vi "Main_18a not correct.vi"() -> ()   [LabVIEW 2020]
uses:
  RB ENUM_face state.ctl
panel:
  out "MAX":i32
  out "total":i32
  out "number of rows":i32
  in  "Example 2":string="2,2,2\n1,2,2\n3,2,2\n2,1,2\n2,3,2\n2,2,1\n2,2,3\n2,2,4\n2,2,6\n1,2,5\n3,2,5\n2,1,5\n2,3,5"
  out "z":i32
  out "x":i32
  out "y":i32
  out "Array":cluster{"facecube":T1[][][]}[](array[cluster])
  out "Answer":i32
  in  "Puzzle":string="8,17,5\n6,17,7\n8,9,2\n13,5,16\n5,3,9\n19,4,10\n5,14,5\n3,5,12\n4,6,13\n11,9,3\n11,2,14\n3,14,10\n12,1,11\n16,16,13\n1,9,10\n11,9,19\n15,15,12\n10,4,6\n4,12,17\n17,6,15\n19,14,13\n9,13,2\n18,8,14\n17,7,15\n10,5,17\n14,8,17\n11,19,13\n13,3,14\n8,5,10\n8,16,6\n10,7,20\n7,17,5\n12,18,13\n4,8,13\n3,13,13\n4,3,11\n4,9,15\n17,6,7\n13,5,14\n3,12,7\n13,18,7\n1,9,11\n17,8,15\n12,8,2\n4,9,6\n3,7,12\n8,13,4\n3,8,7\n14,7,3\n16,7,14\n17,5,12\n13,8,2\n17,5,5\n16,5,13\n5,4,13\n6,1,9\n1,11,10\n5,13,5\n10,17,5\n6,3,9\n15,6,7\n11,15,17\n18,6,12\n8,3,11\n14,7,14\n10,6,18\n12,11,4\n3,7,15\n7,3,10\n18,8,13\n16,11,19\n11,3,11\n3,15,14\n16,14,3\n19,10,8\n8,13,18\n15,10,3\n20,7,12\n13,15,16\n18,10,9\n10,2,7\n16,5,12\n6,10,18\n12,19,13\n6,5,6\n14,2,8\n4,16,9\n6,17,9\n15,6,5\n9,4,3\n11,7,2\n19,9,6\n14,12,2\n15,6,18\n18,13,7\n5,6,6\n20,11,14\n19,10,10\n18,10,6\n6,10,5\n16,10,18\n3,9,7\n13,2,7\n14,9,19\n9,14,19\n7,18,6\n8,9,19\n11,1,13\n15,17,10\n2,12,13\n5,17,14\n18,9,11\n15,18,15\n7,3,11\n10,18,6\n17,15,14\n17,7,8\n7,3,14\n7,11,19\n7,9,3\n17,11,6\n16,3,10\n9,18,16\n13,1,10\n15,12,16\n14,12,20\n11,2,8\n18,5,9\n11,16,3\n18,10,7\n4,12,6\n5,11,18\n3,14,14\n16,4,12\n8,3,4\n6,14,3\n17,9,18\n2,11,7\n19,15,12\n13,17,15\n10,7,3\n1,11,8\n18,12,16\n18,12,9\n7,4,4\n12,2,7\n7,14,15\n15,13,3\n3,7,11\n12,17,10\n17,5,14\n5,18,11\n5,4,11\n4,15,15\n8,19,12\n18,12,10\n9,3,11\n3,14,12\n18,7,16\n10,9,19\n16,3,11\n15,11,17\n18,7,12\n9,8,19\n3,15,12\n17,4,12\n5,16,7\n8,4,5\n2,7,11\n5,15,17\n9,20,12\n5,11,4\n4,5,9\n4,15,11\n14,14,5\n11,3,6\n12,3,15\n5,6,10\n5,9,5\n18,15,12\n4,12,5\n19,9,15\n4,6,11\n1,14,9\n5,16,15\n9,3,7\n16,10,4\n17,12,7\n18,8,7\n14,5,9\n6,6,14\n5,14,15\n6,7,3\n18,15,15\n12,7,17\n5,14,16\n6,11,3\n6,10,16\n3,7,8\n10,7,4\n8,8,3\n11,4,5\n16,13,18\n13,6,4\n10,17,16\n3,16,10\n10,19,13\n15,5,16\n9,19,6\n9,13,4\n17,16,7\n12,4,15\n7,4,15\n18,17,10\n14,17,7\n13,15,19\n4,10,15\n13,18,17\n14,19,10\n18,10,15\n14,18,8\n16,4,13\n17,14,9\n14,17,5\n6,7,4\n5,9,16\n5,14,17\n14,19,11\n6,18,7\n14,9,18\n17,7,16\n4,10,16\n11,13,3\n3,10,16\n8,9,18\n13,3,15\n17,8,6\n3,13,9\n5,17,10\n14,15,3\n15,5,15\n16,17,15\n9,20,8\n8,2,13\n20,8,8\n17,14,12\n5,7,18\n5,10,16\n3,8,11\n3,11,16\n15,7,5\n17,12,18\n10,19,11\n11,2,10\n18,11,6\n5,11,17\n15,10,15\n18,15,9\n7,5,15\n17,8,5\n5,5,6\n17,14,16\n15,11,5\n8,10,19\n3,13,14\n7,3,9\n13,2,8\n17,9,6\n17,16,11\n11,10,18\n12,17,18\n5,3,14\n12,9,2\n5,14,6\n14,15,15\n15,4,9\n8,12,17\n10,9,3\n4,17,9\n1,11,12\n3,14,11\n11,19,9\n12,17,8\n5,5,9\n19,9,12\n16,4,14\n18,10,14\n8,19,13\n11,3,8\n6,6,4\n13,6,18\n6,14,4\n18,6,8\n4,13,15\n11,7,1\n11,7,18\n10,3,7\n14,15,7\n6,16,9\n14,7,19\n12,6,17\n16,12,5\n3,10,7\n7,12,5\n16,10,15\n17,8,11\n10,18,14\n3,11,4\n7,10,19\n10,4,3\n12,16,6\n9,8,1\n10,4,15\n14,4,5\n5,8,16\n8,13,3\n19,10,9\n17,17,13\n4,5,11\n14,5,16\n16,11,17\n17,7,6\n1,10,11\n11,8,16\n4,15,6\n10,19,14\n6,4,9\n18,11,8\n10,4,5\n11,13,19\n13,6,16\n5,10,17\n3,11,5\n18,17,9\n18,14,11\n10,1,7\n15,9,3\n8,6,3\n6,3,12\n12,2,8\n14,16,17\n16,8,4\n15,7,4\n19,15,9\n17,16,9\n7,14,19\n3,10,8\n9,20,13\n8,8,1\n5,12,4\n8,17,15\n17,3,10\n16,8,6\n18,10,5\n15,8,5\n6,12,4\n1,16,10\n15,17,6\n20,11,11\n4,4,14\n9,9,3\n6,15,17\n16,9,17\n12,12,19\n19,8,10\n4,14,17\n9,15,17\n10,3,14\n4,6,7\n2,8,12\n13,2,11\n7,11,2\n10,19,7\n15,10,2\n6,13,3\n11,10,20\n6,12,18\n15,18,13\n10,8,2\n13,5,5\n11,2,9\n6,17,14\n6,8,5\n14,14,16\n6,8,16\n3,12,16\n8,17,18\n12,2,11\n3,15,11\n10,11,2\n11,17,12\n9,15,3\n6,16,17\n18,6,6\n16,12,16\n7,18,12\n17,15,4\n9,12,18\n17,6,6\n11,8,19\n12,8,3\n20,9,14\n4,12,16\n20,11,10\n4,15,8\n4,7,9\n16,7,5\n10,9,18\n2,11,12\n4,13,16\n9,2,10\n16,7,18\n17,11,16\n6,15,4\n7,18,7\n6,9,19\n8,15,4\n5,16,14\n2,10,7\n8,12,4\n14,18,13\n12,14,17\n15,11,19\n6,13,16\n14,7,18\n19,11,7\n6,17,16\n10,11,3\n7,20,13\n10,18,7\n8,17,6\n4,7,16\n8,3,15\n2,10,9\n5,3,13\n17,10,15\n9,4,6\n8,19,11\n9,16,4\n14,8,19\n13,12,15\n4,13,17\n14,16,5\n5,6,16\n14,13,17\n18,7,13\n12,3,6\n6,4,14\n10,4,9\n3,10,6\n8,19,9\n11,7,19\n19,12,14\n18,9,10\n16,10,17\n16,6,16\n17,15,15\n7,18,11\n1,10,12\n12,4,13\n8,5,5\n20,10,12\n9,18,8\n18,13,9\n8,17,4\n18,7,6\n7,13,4\n15,17,14\n11,17,17\n4,11,16\n7,5,17\n8,15,17\n14,18,6\n15,12,3\n2,7,13\n11,5,5\n19,14,11\n15,18,9\n11,18,5\n7,6,6\n10,11,19\n8,14,3\n6,13,17\n12,5,15\n16,9,3\n3,5,6\n10,4,16\n14,13,19\n3,6,12\n9,15,14\n17,13,7\n7,19,11\n8,14,16\n3,17,12\n9,11,18\n18,14,7\n17,17,9\n8,13,2\n4,16,15\n11,15,4\n8,4,9\n13,6,17\n4,7,12\n13,3,10\n6,5,9\n5,6,5\n15,14,5\n11,4,6\n4,17,13\n3,11,11\n16,13,5\n12,9,1\n13,9,18\n8,17,9\n5,11,15\n16,14,5\n13,11,19\n10,16,17\n9,12,3\n3,12,10\n6,9,4\n5,13,15\n11,6,18\n16,4,9\n7,12,3\n18,12,6\n10,16,18\n14,6,18\n4,5,7\n6,8,18\n15,10,18\n8,3,13\n10,5,18\n3,6,15\n14,6,16\n14,6,17\n12,10,3\n2,14,12\n18,5,10\n15,9,17\n8,6,18\n3,16,14\n10,13,4\n10,15,19\n4,8,17\n13,6,5\n3,6,10\n12,20,10\n11,6,4\n18,4,11\n17,9,11\n15,4,13\n9,17,5\n6,3,11\n11,19,6\n17,6,14\n7,7,18\n8,10,2\n9,3,15\n4,16,13\n11,5,15\n3,6,13\n8,15,18\n14,3,14\n6,5,14\n5,12,18\n8,3,12\n15,4,16\n6,6,15\n16,16,9\n15,3,14\n8,14,18\n10,17,6\n5,9,6\n15,8,16\n18,6,5\n15,13,4\n15,16,5\n10,7,5\n9,7,18\n16,3,13\n4,8,4\n11,11,19\n17,13,12\n17,11,15\n4,13,14\n10,2,6\n4,10,4\n10,3,6\n9,16,17\n8,1,9\n14,20,9\n3,7,14\n8,18,16\n3,11,14\n16,14,15\n3,10,9\n17,12,12\n3,14,5\n10,16,3\n5,15,13\n15,16,7\n12,16,19\n2,12,11\n2,13,10\n13,18,14\n16,15,18\n2,10,15\n2,8,8\n6,7,6\n13,5,17\n6,4,15\n9,17,6\n5,16,13\n11,5,18\n7,17,10\n17,6,5\n14,4,12\n8,12,20\n2,15,10\n18,6,13\n12,19,16\n19,7,5\n19,9,14\n10,13,18\n6,11,19\n10,14,3\n19,7,11\n7,18,16\n14,9,2\n12,4,5\n15,14,6\n5,9,17\n11,14,2\n15,13,18\n16,16,8\n2,5,9\n2,8,10\n16,5,6\n6,18,10\n12,18,15\n4,14,12\n15,8,17\n18,9,9\n11,10,1\n12,3,3\n9,19,9\n8,5,13\n20,14,12\n16,5,15\n1,12,10\n19,15,11\n13,17,10\n12,2,5\n3,5,10\n7,6,5\n5,7,4\n9,6,18\n16,17,12\n7,8,19\n17,11,12\n10,18,15\n13,16,15\n2,12,14\n8,12,2\n14,18,7\n17,5,9\n3,13,5\n10,14,19\n3,8,13\n16,15,3\n11,6,20\n3,14,8\n14,8,18\n7,17,12\n4,13,5\n17,7,5\n8,7,17\n14,4,6\n17,12,4\n13,3,6\n10,12,3\n9,21,11\n17,11,13\n2,16,13\n7,5,3\n14,16,16\n17,15,6\n14,3,13\n11,3,13\n16,16,15\n13,2,13\n17,14,15\n12,2,15\n17,14,11\n10,14,4\n6,8,4\n16,7,15\n11,4,17\n17,17,11\n12,4,17\n6,9,15\n12,9,20\n16,11,5\n18,5,7\n8,11,18\n15,12,6\n12,13,3\n7,15,3\n5,11,3\n11,16,8\n16,17,14\n4,8,7\n14,5,7\n4,13,18\n15,17,7\n16,15,17\n14,20,11\n10,6,14\n12,19,10\n13,3,16\n13,18,8\n13,19,10\n10,10,3\n9,2,8\n6,16,16\n6,16,7\n13,17,5\n3,8,12\n12,13,17\n13,19,12\n19,13,8\n6,10,17\n16,16,7\n7,14,6\n5,15,6\n13,1,12\n7,3,13\n11,17,6\n13,15,3\n10,2,12\n14,2,13\n19,11,6\n8,8,17\n4,6,6\n4,16,10\n4,5,12\n14,19,14\n17,15,16\n11,15,18\n10,15,3\n8,2,10\n15,9,8\n17,13,16\n2,13,14\n15,7,6\n10,12,20\n4,17,14\n12,6,16\n18,7,7\n5,9,4\n16,15,7\n18,16,10\n10,2,10\n13,17,17\n15,6,12\n10,7,2\n11,0,12\n13,2,6\n17,9,5\n10,16,5\n19,10,13\n7,11,16\n5,17,13\n8,18,13\n15,7,19\n3,12,8\n7,18,15\n12,17,3\n16,5,16\n9,16,16\n14,5,15\n8,2,9\n7,16,7\n12,5,16\n19,8,15\n17,10,16\n9,5,6\n12,7,4\n3,4,9\n11,14,19\n12,12,1\n15,12,4\n16,12,17\n18,10,12\n19,12,6\n15,8,15\n12,19,14\n3,8,6\n14,2,12\n11,5,4\n10,5,3\n9,11,3\n7,12,19\n3,5,7\n20,7,11\n15,3,12\n13,4,9\n13,14,2\n17,13,14\n16,4,11\n10,3,17\n15,16,8\n18,16,8\n4,14,14\n11,19,8\n5,11,6\n9,3,16\n10,17,7\n13,9,19\n5,13,8\n12,4,4\n8,13,1\n7,2,11\n6,6,5\n9,5,3\n12,14,3\n14,3,11\n10,6,4\n8,16,18\n10,18,17\n9,7,2\n6,5,8\n10,2,13\n17,8,16\n6,3,10\n7,13,18\n8,18,14\n4,9,17\n12,7,19\n3,12,11\n16,16,14\n4,14,13\n9,5,5\n4,6,16\n7,16,16\n12,15,17\n19,16,11\n8,9,16\n1,13,13\n16,15,5\n2,11,8\n6,2,12\n9,5,15\n12,2,13\n8,13,19\n15,5,7\n7,19,9\n7,1,8\n17,8,4\n5,5,4\n5,4,12\n11,12,3\n8,15,3\n16,16,12\n16,13,17\n5,6,8\n10,10,2\n4,16,14\n10,8,20\n3,9,16\n5,12,5\n7,16,6\n18,6,14\n6,5,17\n2,7,8\n16,17,11\n12,3,12\n11,4,16\n17,11,5\n13,4,11\n15,6,8\n6,10,6\n11,1,10\n10,19,12\n3,14,13\n12,18,9\n7,15,5\n10,3,9\n10,8,18\n16,14,4\n20,9,9\n10,15,2\n10,5,16\n10,17,4\n14,11,2\n15,9,4\n15,3,9\n15,6,17\n2,9,11\n7,13,17\n6,17,15\n16,12,4\n16,5,7\n11,5,17\n5,12,7\n10,3,13\n6,10,4\n17,10,4\n6,4,10\n14,18,14\n12,18,10\n13,18,6\n15,6,13\n15,16,12\n16,6,12\n17,10,7\n17,10,5\n1,9,12\n3,9,5\n17,15,7\n13,13,4\n4,5,13\n15,12,2\n13,4,4\n15,13,17\n19,12,10\n15,18,7\n12,17,17\n16,7,4\n19,7,12\n3,12,5\n11,19,12\n10,20,9\n13,15,18\n18,6,11\n9,1,10\n12,8,20\n18,13,10\n2,12,15\n3,6,11\n14,8,16\n7,10,5\n4,13,6\n10,14,1\n7,12,18\n10,18,11\n2,11,13\n6,6,6\n17,4,8\n13,4,16\n5,14,9\n18,12,5\n4,12,12\n18,15,11\n12,17,4\n17,7,11\n12,17,15\n13,10,1\n2,15,9\n4,10,5\n6,14,6\n15,7,7\n6,16,12\n15,9,2\n12,2,12\n9,4,5\n3,14,7\n9,15,5\n4,7,8\n8,16,17\n19,6,9\n19,8,7\n13,3,9\n14,13,15\n7,17,14\n8,4,12\n13,18,9\n6,5,15\n17,5,6\n13,13,3\n13,17,13\n13,6,2\n11,3,9\n3,8,14\n7,4,8\n4,14,6\n8,5,18\n13,7,18\n13,7,3\n14,11,17\n7,5,16\n13,3,12\n19,12,15\n14,3,5\n17,11,18\n9,3,10\n15,7,3\n2,9,12\n6,18,9\n3,6,9\n13,19,7\n18,11,7\n3,15,8\n2,12,12\n16,15,11\n4,4,11\n6,7,11\n1,10,13\n15,3,11\n14,18,10\n6,9,18\n18,9,15\n12,19,11\n7,6,7\n3,12,18\n3,11,9\n14,17,6\n16,16,11\n18,14,14\n8,20,11\n18,6,7\n15,6,16\n5,9,3\n14,2,14\n10,7,18\n7,4,17\n20,6,9\n15,5,10\n15,4,12\n20,10,15\n6,12,2\n10,4,4\n5,15,15\n5,16,10\n6,11,2\n10,13,2\n7,15,4\n15,16,4\n16,5,8\n4,6,15\n8,5,14\n4,17,12\n6,14,5\n11,17,7\n15,14,15\n17,12,5\n6,18,13\n16,17,9\n7,7,16\n4,6,9\n7,10,3\n16,14,12\n19,12,12\n15,17,9\n13,2,12\n6,9,3\n12,3,9\n15,14,3\n14,14,19\n14,8,3\n9,8,18\n4,13,7\n10,4,8\n8,1,7\n5,5,13\n14,3,16\n6,20,9\n6,15,18\n5,14,18\n19,9,8\n5,2,12\n16,8,15\n10,3,8\n13,15,4\n8,16,3\n13,13,2\n14,18,12\n16,5,14\n11,14,18\n5,7,5\n8,9,20\n9,8,3\n16,16,6\n13,20,9\n11,18,14\n15,13,5\n11,14,17\n12,17,6\n10,17,15\n6,8,15\n2,7,12\n12,20,13\n9,14,17\n12,16,5\n10,19,6\n7,7,4\n1,11,11\n19,6,10\n15,14,4\n19,13,12\n4,7,6\n9,2,12\n9,19,15\n18,14,16\n11,10,2\n13,16,4\n17,12,15\n2,10,10\n2,13,13\n5,10,3\n10,16,7\n11,19,10\n17,14,8\n12,12,20\n7,5,8\n11,8,20\n5,15,8\n3,9,8\n13,5,13\n17,15,10\n14,11,19\n15,5,4\n15,3,8\n15,4,6\n4,15,14\n17,11,17\n12,6,15\n3,16,7\n4,11,5\n13,10,3\n7,14,3\n6,17,12\n14,16,4\n4,16,12\n4,14,5\n14,19,9\n19,13,9\n10,10,19\n11,11,1\n18,16,12\n17,17,8\n10,12,2\n7,18,8\n1,8,12\n19,8,6\n4,6,8\n13,14,17\n20,10,8\n19,7,7\n12,3,14\n2,9,8\n5,17,11\n11,8,2\n7,18,9\n8,7,3\n9,15,18\n10,6,16\n7,16,3\n15,8,18\n11,14,3\n17,13,6\n11,8,18\n14,5,5\n17,16,14\n17,13,4\n9,7,17\n13,5,6\n14,3,12\n3,13,16\n11,3,7\n16,10,16\n11,16,4\n7,3,15\n5,16,11\n20,9,10\n18,8,9\n19,8,8\n20,9,13\n11,16,16\n15,11,2\n1,13,12\n14,13,4\n12,18,11\n14,16,3\n11,5,11\n17,7,13\n15,11,18\n7,17,9\n5,5,14\n11,9,2\n4,7,14\n7,17,15\n5,12,17\n3,8,15\n18,10,16\n15,4,11\n12,5,6\n19,11,11\n11,18,17\n18,13,16\n7,4,7\n7,5,6\n13,10,19\n13,18,10\n16,15,16\n5,7,15\n12,12,2\n2,14,8\n20,9,11\n4,7,11\n5,11,12\n16,16,10\n3,17,9\n2,9,9\n17,18,9\n3,12,15\n5,3,11\n15,4,15\n20,10,14\n19,13,11\n5,13,18\n17,9,4\n13,12,17\n3,15,13\n14,10,6\n16,16,5\n5,8,17\n15,3,6\n18,15,10\n15,6,6\n18,11,14\n17,12,13\n4,6,14\n5,14,3\n15,5,6\n11,15,3\n12,2,9\n14,3,15\n17,12,16\n15,17,13\n13,12,1\n14,3,10\n18,9,14\n12,17,11\n16,11,15\n18,8,6\n3,12,6\n3,9,6\n7,16,8\n16,12,15\n18,8,10\n4,5,10\n12,19,7\n14,2,9\n8,7,6\n12,3,11\n4,7,7\n9,18,14\n4,6,5\n11,17,16\n8,19,10\n12,8,19\n3,17,13\n15,12,18\n4,4,13\n10,19,8\n16,8,17\n9,7,16\n19,14,9\n9,8,2\n16,8,13\n7,5,14\n7,6,4\n18,11,10\n6,4,5\n18,7,14\n18,11,13\n9,6,3\n8,16,15\n7,8,3\n12,9,3\n9,19,7\n8,6,16\n10,4,17\n17,4,14\n11,13,18\n6,8,17\n3,7,17\n16,4,8\n2,10,8\n5,18,8\n9,3,6\n18,9,5\n9,15,19\n3,16,9\n7,6,17\n7,16,17\n12,11,19\n12,10,2\n4,7,10\n6,19,13\n19,11,10\n9,10,1\n12,14,4\n4,9,4\n18,16,9\n5,3,8\n9,18,4\n3,13,6\n16,15,14\n13,8,19\n12,16,14\n8,10,15\n11,21,12\n5,15,5\n8,9,15\n18,11,5\n16,17,8\n10,17,17\n11,8,3\n7,19,12\n14,16,8\n17,15,12\n11,11,4\n7,6,19\n3,16,12\n17,5,10\n11,3,16\n8,15,14\n8,15,5\n2,9,13\n5,11,5\n4,4,8\n12,5,17\n7,5,7\n6,19,11\n4,7,4\n17,9,7\n15,7,16\n9,14,3\n14,4,15\n16,7,17\n3,12,9\n17,9,16\n8,18,10\n11,16,5\n10,18,8\n14,5,6\n12,15,16\n10,6,19\n14,7,17\n2,14,11\n8,5,8\n16,9,4\n8,3,7\n8,3,14\n19,9,13\n6,8,3\n17,14,17\n13,3,13\n4,13,4\n3,10,14\n17,16,12\n17,5,11\n12,3,10\n15,8,3\n17,9,14\n14,7,4\n5,9,18\n10,2,9\n13,4,7\n7,15,17\n11,13,20\n8,18,7\n12,13,20\n17,16,13\n10,6,2\n3,6,5\n7,2,13\n12,4,16\n14,15,18\n12,9,17\n8,12,18\n7,10,2\n17,3,8\n9,3,9\n14,9,3\n10,3,10\n14,6,5\n16,14,10\n6,3,13\n9,19,12\n19,9,11\n9,9,19\n17,15,13\n19,6,13\n10,3,12\n15,4,14\n10,5,5\n6,12,16\n10,11,18\n4,9,5\n19,15,8\n4,15,7\n14,16,14\n12,1,9\n9,14,2\n12,15,3\n14,10,17\n15,15,17\n14,4,10\n3,13,12\n17,17,10\n9,17,4\n3,9,11\n11,15,13\n20,11,8\n18,13,13\n3,11,8\n14,3,7\n18,11,12\n19,14,8\n18,13,6\n10,16,16\n9,1,12\n5,8,13\n11,2,13\n2,15,8\n11,3,14\n8,17,14\n8,6,6\n5,13,4\n5,15,4\n4,3,7\n14,17,14\n12,15,2\n13,5,4\n14,15,4\n15,14,16\n19,12,9\n19,8,11\n7,11,3\n3,5,13\n6,13,19\n15,13,6\n11,6,17\n18,8,8\n11,18,10\n10,12,18\n2,10,12\n18,9,17\n18,7,8\n7,16,11\n9,20,11\n17,13,17\n9,14,1\n4,4,12\n6,19,10\n2,9,14\n18,11,11\n18,5,13\n3,7,13\n13,12,2\n13,17,6\n2,7,9\n18,8,11\n4,16,11\n7,7,5\n14,17,16\n12,3,5\n11,17,18\n15,16,16\n9,13,19\n17,14,14\n6,17,6\n13,4,5\n5,8,18\n9,11,20\n17,10,8\n8,16,2\n17,7,7\n14,14,17\n15,7,14\n14,10,19\n6,11,5\n15,8,4\n9,3,14\n5,14,4\n4,11,4\n15,16,11\n7,16,14\n8,18,12\n17,12,6\n6,9,17\n13,15,17\n4,4,9\n8,7,18\n12,19,9\n16,14,17\n2,7,7\n7,14,18\n18,12,15\n5,17,9\n6,2,9\n12,19,15\n5,7,17\n16,15,15\n13,3,11\n8,2,11\n11,4,8\n10,12,21\n9,15,16\n3,7,9\n10,2,11\n4,8,6\n17,10,6\n11,3,17\n4,11,18\n11,4,3\n4,11,8\n18,5,8\n12,13,2\n14,4,4\n13,11,18\n8,14,2\n6,7,16\n20,11,13\n12,3,7\n4,11,10\n6,3,6\n12,18,7\n8,5,11\n15,2,11\n17,5,7\n18,14,9\n9,4,11\n13,11,3\n10,19,10\n18,14,8\n16,11,4\n10,4,11\n10,8,19\n13,18,5\n10,9,1\n13,20,10\n6,8,6\n10,14,2\n18,8,5\n9,14,18\n3,8,8\n16,9,16\n17,8,14\n9,6,16\n7,9,20\n3,13,11\n17,8,13\n18,10,4\n16,6,9\n12,19,8\n6,15,6\n8,8,4\n7,14,4\n13,17,14\n19,6,6\n4,17,11\n8,17,16\n12,9,19\n2,11,11\n19,8,13\n6,5,5\n9,17,16\n14,4,9\n17,8,9\n4,13,9\n2,8,13\n17,4,10\n13,8,16\n2,13,11\n5,5,11\n15,9,19\n11,15,19\n7,17,18\n7,3,7\n13,16,16\n8,17,12\n15,2,14\n9,9,2\n7,4,13\n7,18,14\n5,16,5\n17,16,8\n11,1,7\n4,11,13\n18,11,9\n4,15,10\n2,7,10\n12,10,18\n7,10,16\n14,3,6\n20,10,11\n4,8,11\n6,15,5\n3,12,13\n5,4,10\n2,9,7\n16,5,9\n13,5,3\n15,7,17\n6,16,11\n9,18,15\n10,20,10\n13,8,18\n19,10,12\n5,6,17\n17,10,3\n15,11,3\n18,12,11\n13,4,6\n13,14,16\n2,12,10\n6,14,18\n15,16,6\n10,18,10\n4,14,16\n3,13,7\n13,8,20\n10,18,5\n12,2,10\n18,5,11\n15,2,6\n13,7,2\n10,3,15\n10,15,16\n4,6,12\n20,12,7\n8,3,10\n16,4,10\n20,13,8\n17,3,12\n13,11,4\n8,3,8\n7,3,6\n5,17,8\n18,13,11\n14,11,16\n5,11,16\n11,16,6\n16,9,5\n4,3,9\n14,4,16\n5,10,4\n7,2,10\n14,4,8\n14,17,9\n4,5,15\n15,15,5\n6,17,8\n5,3,12\n3,14,9\n8,12,19\n5,7,11\n18,7,15\n9,5,2\n13,10,17\n7,9,18\n19,7,13\n3,7,6\n13,9,2\n4,10,13\n10,14,17\n3,12,12\n12,7,18\n16,6,7\n15,8,19\n9,15,4\n12,7,2\n14,13,18\n6,4,11\n3,7,5\n18,9,13\n17,3,11\n5,4,15\n9,16,3\n13,10,2\n16,19,10\n19,14,10\n13,2,14\n9,3,13\n12,18,12\n15,18,12\n10,20,14\n6,7,18\n13,8,3\n6,11,20\n8,4,10\n11,3,10\n5,6,13\n8,2,12\n2,9,10\n3,12,14\n2,12,7\n18,6,15\n15,13,19\n16,15,9\n17,5,8\n7,6,18\n7,2,7\n19,7,9\n17,6,12\n6,19,14\n5,16,17\n6,10,3\n7,12,4\n17,15,11\n12,8,18\n2,14,13\n5,8,6\n15,4,10\n7,7,17\n19,9,9\n16,14,8\n16,7,13\n11,10,3\n14,11,1\n16,15,12\n5,15,7\n7,3,8\n12,3,13\n11,3,15\n9,3,5\n13,2,10\n19,11,9\n11,12,20\n8,8,2\n7,9,19\n19,13,14\n18,9,6\n18,15,14\n5,6,14\n20,5,9\n8,4,15\n8,16,5\n2,6,11\n8,4,4\n6,19,9\n7,18,10\n14,8,4\n9,18,7\n9,6,19\n9,5,16\n18,15,7\n16,16,16\n8,12,3\n5,16,9\n5,6,15\n15,6,4\n8,2,14\n9,13,1\n2,14,7\n11,16,2\n9,18,6\n18,9,16\n17,15,8\n6,13,14\n14,4,11\n9,12,2\n11,16,18\n9,4,9\n15,15,6\n9,8,17\n5,12,6\n16,8,3\n15,14,2\n6,18,14\n18,16,14\n14,7,6\n16,3,9\n15,6,14\n10,15,18\n7,5,4\n12,3,16\n9,6,14\n6,18,15\n18,15,8\n6,15,7\n16,3,8\n2,13,8\n9,16,5\n8,7,16\n18,11,17\n17,9,17\n17,8,17\n17,12,17\n16,6,6\n8,11,3\n5,13,14\n8,2,8\n15,17,11\n5,6,9\n2,11,9\n11,2,11\n5,18,12\n18,16,11\n6,9,8\n12,5,4\n1,8,8\n6,14,17\n12,8,1\n13,3,7\n2,10,13\n7,13,3\n17,14,13\n15,18,14\n7,17,7\n13,15,2\n9,2,13\n6,2,10\n6,14,14\n15,14,12\n8,2,15\n13,11,2\n4,15,13\n18,12,14\n16,17,7\n20,10,9\n16,15,6\n12,11,3\n6,18,12\n11,4,4\n18,11,16\n17,12,9\n3,8,5\n7,4,6\n13,4,13\n18,9,7\n15,5,12\n2,13,12\n14,3,9\n3,6,8\n16,8,11\n11,12,18\n19,12,13\n16,15,4\n13,16,6\n4,9,7\n12,9,5\n15,7,18\n15,10,5\n19,5,10\n10,2,8\n10,4,14\n17,4,11\n19,14,12\n3,11,13\n8,18,9\n1,10,9\n6,4,7\n12,7,3\n2,15,11\n13,19,11\n14,17,10\n2,5,12\n11,20,10\n4,7,17\n10,17,8\n7,11,18\n4,10,17\n13,12,20\n7,8,4\n19,13,13\n4,5,8\n13,6,19\n5,12,3\n5,16,6\n13,4,12\n9,11,2\n15,15,2\n5,16,8\n8,3,16\n13,4,15\n14,12,4\n13,16,5\n14,15,5\n4,7,5\n6,4,13\n11,18,8\n12,17,5\n7,2,9\n14,2,11\n10,10,20\n9,10,20\n17,15,9\n12,14,18\n8,11,19\n19,7,14\n10,13,19\n12,10,19\n6,20,11\n5,8,15\n7,2,8\n9,12,20\n8,13,16\n2,14,6\n3,10,5\n16,7,6\n7,2,12\n6,16,6\n13,7,4\n14,9,17\n9,19,8\n3,5,11\n17,4,9\n16,15,8\n10,5,6\n9,1,9\n6,4,16\n19,12,11\n6,9,5\n11,17,10\n10,19,15\n9,15,2\n3,17,8\n20,13,11\n15,4,7\n7,17,16\n8,16,7\n18,9,12\n3,10,12\n4,14,10\n4,5,14\n4,6,10\n15,17,15\n11,11,3\n12,2,14\n9,7,3\n9,3,8\n13,20,13\n4,12,4\n8,4,7\n16,6,10\n19,10,7\n6,3,15\n5,7,16\n9,1,15\n8,1,11\n4,8,15\n8,11,20\n8,16,4\n13,1,9\n11,6,3\n6,11,4\n15,16,14\n5,4,14\n10,20,11\n14,2,10\n19,11,12\n18,12,13\n7,10,18\n3,14,15\n4,12,9\n5,8,4\n8,20,9\n13,5,15\n14,19,13\n18,9,8\n10,12,19\n4,13,11\n4,18,14\n16,5,10\n12,4,6\n16,8,8\n6,5,4\n11,4,18\n7,4,9\n9,5,17\n17,9,15\n16,12,12\n16,18,9\n5,5,10\n3,5,8\n4,10,14\n6,15,16\n8,1,10\n17,14,10\n15,10,4\n11,9,20\n5,7,3\n13,7,16\n12,10,20\n18,10,10\n4,10,10\n7,4,3\n15,9,18\n11,12,4\n8,10,17\n4,19,10\n8,19,8\n16,9,2\n11,2,7\n11,7,17\n10,8,3\n9,11,19\n7,13,2\n11,17,4\n10,12,1\n5,5,8\n13,13,19\n16,18,15\n6,16,8\n15,17,16\n15,10,17\n13,15,15\n11,3,12\n13,12,18\n7,16,5\n12,11,1\n19,7,10\n7,3,12\n19,12,7\n18,16,7\n13,14,3\n15,13,2\n8,6,4\n8,6,15\n5,14,11\n3,9,14\n8,5,4\n14,12,16\n19,8,12\n10,7,19\n9,16,18\n11,18,13\n15,16,17\n3,9,13\n10,13,1\n16,13,4\n8,11,1\n14,5,3\n12,6,18\n18,8,15\n11,18,11\n4,14,8\n5,12,15\n2,8,9\n3,10,13\n6,12,17\n3,6,14\n8,7,4\n16,8,18\n4,5,5\n4,8,9\n16,19,11\n13,3,8\n6,6,17\n4,12,13\n8,17,17\n10,13,3\n16,16,4\n12,6,5\n7,19,13\n18,14,12\n14,6,3\n17,7,12\n17,16,10\n2,12,9\n1,12,12\n11,13,17\n15,17,8\n11,3,5\n14,4,14\n9,4,13\n12,16,17\n5,17,7\n18,4,10\n12,18,5\n3,15,10\n9,10,19\n6,10,2\n10,6,1\n6,12,3\n13,4,17\n15,15,16\n5,15,12\n15,15,14\n11,2,5\n12,5,3\n14,18,11\n15,16,15\n11,19,7\n3,11,7\n5,9,14\n9,1,13\n15,18,11\n14,12,3\n11,20,9\n2,13,15\n4,18,12\n10,4,7\n19,13,10\n11,20,12\n9,8,16\n12,18,14\n9,18,13\n12,16,15\n17,5,13\n11,2,6\n9,4,17\n7,17,13\n11,6,15\n18,13,14\n9,17,15\n12,11,2\n16,17,13\n6,16,4\n14,14,3\n19,10,11\n16,6,5\n10,18,4\n6,13,2\n18,9,4\n10,9,2\n13,16,17\n13,18,15\n7,17,11\n6,13,4\n1,12,13\n11,1,12\n18,14,10\n7,19,14\n10,3,16\n10,21,12\n15,19,10\n9,13,3\n13,7,17\n8,11,2\n6,5,7\n6,13,5\n13,17,8\n15,4,8\n19,10,6\n2,11,6\n10,19,9\n5,4,7\n10,17,13\n6,13,18\n8,7,19\n2,12,8\n9,2,6\n12,6,19\n13,12,3\n7,4,11\n3,13,17\n10,2,5\n20,7,8\n14,4,7\n13,17,4\n14,18,15\n15,6,15\n8,17,8\n3,9,9\n17,18,7\n5,7,7\n3,11,12\n17,6,13\n4,11,7\n17,8,18\n5,14,14\n5,6,4\n6,18,11\n17,3,13\n3,13,8\n5,7,6\n1,13,10\n5,13,16\n19,7,8\n4,11,17\n6,17,13\n15,17,5\n18,13,8\n18,8,16\n1,8,13\n4,9,12\n12,15,18\n7,13,5\n9,18,17\n11,6,16\n13,4,14\n9,4,4\n10,17,14\n13,14,18\n12,15,19\n6,12,6\n7,19,10\n1,12,9\n20,10,13\n14,14,15\n12,15,4\n4,12,15\n5,10,18\n10,8,17\n6,6,3\n3,10,10\n5,18,7\n7,12,17\n8,15,2\n12,14,20\n11,16,17\n4,14,15\n13,20,8\n4,11,14\n7,16,15\n9,19,14\n9,6,20\n3,16,8\n10,1,8\n11,13,1\n14,1,11\n16,18,10\n1,11,9\n14,20,10\n9,19,13\n10,20,12\n3,14,16\n19,6,11\n18,11,15\n19,13,7\n8,18,6\n17,6,16\n16,13,15\n14,15,2\n13,1,8\n6,4,8\n17,6,10\n1,8,10\n15,16,13\n8,19,6\n2,8,11\n7,10,1\n4,16,6\n19,10,15\n19,16,9\n9,10,18\n16,17,6\n16,10,19\n12,1,10\n15,5,5\n2,6,8\n19,8,14\n4,18,11\n10,11,1\n10,21,10\n6,6,16\n5,5,7\n9,5,18\n8,10,3\n12,18,16\n9,2,7\n9,18,5\n5,4,6\n10,11,20\n9,19,11\n12,19,12\n3,11,10\n15,3,13\n7,17,6\n20,11,9\n11,8,17\n11,11,2\n7,4,10\n18,10,8\n13,13,18\n6,8,19\n18,14,15\n6,19,12\n15,12,5\n18,7,9\n8,12,1\n18,6,10\n3,12,4\n10,13,20\n17,15,5\n3,7,7\n7,14,2\n8,4,16\n11,10,21\n11,12,2\n14,19,12\n2,12,6\n16,10,8\n8,17,7\n6,7,5\n11,12,1\n7,13,16\n3,5,14\n12,20,8\n2,10,14\n4,12,7\n8,16,16\n7,4,16\n8,19,16\n9,1,11\n2,10,11\n10,12,17\n19,11,13\n17,14,6\n11,17,15\n3,15,9\n13,19,8\n6,17,10\n12,3,8\n4,4,10\n16,18,6\n6,16,5\n14,4,13\n7,3,17\n16,14,7\n2,16,12\n5,12,16\n6,17,11\n7,10,15\n15,11,4\n10,16,4\n19,11,14\n4,16,8\n6,9,2\n6,16,15\n18,14,6\n7,1,10\n6,5,13\n17,13,15\n20,13,14\n8,9,3\n16,14,11\n17,13,8\n4,17,10\n2,14,9\n8,3,9\n6,15,15\n19,6,8\n4,4,7\n16,3,14\n9,14,16\n4,10,7\n13,3,17\n16,9,18\n9,2,14\n5,17,5\n14,6,2\n15,2,13\n14,17,15\n7,16,12\n10,4,10\n14,19,8\n9,17,7\n6,9,6\n9,12,19\n12,4,18\n15,11,6\n14,5,17\n17,13,10\n9,19,10\n13,2,9\n12,13,19\n15,2,12\n8,14,4\n5,17,12\n19,9,10\n12,6,3\n15,3,5\n9,6,5\n4,12,8\n12,13,18\n8,5,16\n8,4,14\n13,11,20\n14,13,2\n7,12,7\n9,1,7\n15,16,9\n9,9,20\n5,15,14\n12,10,1\n14,17,8\n8,11,17\n10,18,13\n9,4,7\n14,18,9\n12,19,5\n12,1,8\n9,13,18\n5,7,12\n18,6,16\n3,8,9\n18,15,17\n1,10,14\n12,16,4\n14,7,16\n18,10,11\n7,1,13\n14,7,2\n18,13,15\n16,13,16\n11,5,3\n9,5,4\n14,12,18\n12,13,1\n18,15,13\n2,6,10\n4,17,6\n12,1,12\n4,16,7\n12,16,16\n8,18,15\n14,10,18\n9,9,0\n10,1,13\n9,6,4\n12,6,9\n7,7,3\n9,17,14\n17,14,7\n5,18,9\n12,0,11\n16,11,18\n7,14,16\n14,10,3\n13,12,4\n1,11,6\n13,18,11\n3,6,7\n3,15,7\n3,16,13\n19,12,8\n11,15,6\n12,4,8\n8,7,2\n8,10,18\n3,4,13\n7,6,14\n6,12,5\n20,8,12\n3,9,15\n13,14,4\n16,5,5\n5,4,8\n18,15,6\n7,15,18\n7,13,19\n11,8,4\n12,12,17\n14,5,8\n6,7,2\n14,9,20\n16,10,3\n19,11,8\n13,16,18\n15,4,17\n20,12,9\n11,18,16\n5,10,19\n1,9,13\n10,6,17\n3,9,12\n12,17,7\n16,11,6\n5,17,15\n18,13,12\n3,15,15\n10,3,11\n16,5,4\n20,14,11\n5,10,14\n13,17,16\n12,1,13\n10,4,13\n5,5,16\n11,8,1\n16,4,15\n16,17,16\n6,19,8\n11,6,2\n4,18,10\n6,6,7\n14,11,18\n17,10,18\n11,4,13\n14,12,17\n5,16,12\n2,9,6\n12,4,14\n1,14,11\n13,17,3\n5,18,10\n13,15,6\n11,1,9\n11,20,11\n17,10,14\n14,11,3\n14,9,4\n4,3,8\n14,12,5\n12,12,4\n2,6,9\n8,14,19\n4,7,13\n14,12,19\n4,14,7\n18,6,9\n11,12,17\n13,6,3\n12,7,16\n11,2,15\n18,7,5\n5,9,19\n1,8,9\n12,14,16\n5,15,16\n16,18,13\n11,18,9\n15,9,15\n7,5,13\n17,6,8\n17,7,10\n11,18,15\n10,7,1\n2,8,6\n11,13,2\n5,6,11\n7,16,10\n6,5,10\n7,8,2\n8,6,19\n3,13,10\n18,11,4\n17,3,15\n17,11,8\n9,16,6\n15,3,15\n8,5,17\n7,15,8\n15,13,16\n17,4,13\n15,9,16\n16,12,11\n17,12,11\n6,15,13\n2,8,15\n17,7,14\n8,4,6\n17,11,3\n11,20,8\n11,17,14\n8,8,19\n1,12,14\n14,17,11\n7,16,4\n12,14,19\n11,15,20\n8,5,9\n12,11,17\n16,14,6\n11,5,16\n17,9,3\n16,11,16\n3,7,10\n15,3,7\n13,12,5\n7,14,17\n20,12,12\n11,15,2\n3,11,15\n6,12,7\n7,14,5\n17,13,18\n8,5,6\n7,17,4\n4,9,16\n15,18,6\n14,17,17\n10,14,18\n9,4,10\n16,6,11\n11,18,7\n17,12,14\n13,19,6\n14,14,4\n10,20,13\n6,5,11\n7,12,2\n8,15,16\n3,10,11\n4,11,15\n4,9,14\n4,9,10\n10,5,19\n9,2,11\n15,10,19\n10,18,9\n9,9,18\n16,14,16\n4,13,3\n19,11,15\n19,13,16\n16,6,14\n7,2,14\n8,19,7\n16,4,7\n12,11,20\n16,12,18\n10,8,4\n10,5,15\n20,8,13\n4,18,7\n16,6,15\n14,11,4\n10,2,16\n8,8,20\n14,9,16\n7,6,3\n4,8,14\n10,20,8\n7,13,8\n7,17,17\n14,17,12\n2,8,7\n14,2,6\n15,14,17\n4,8,10\n18,5,12\n5,5,15\n11,7,4\n6,18,8\n17,8,3\n7,6,2\n5,14,7\n9,1,14\n10,11,5\n13,18,13\n1,7,12\n8,4,17\n8,18,11\n17,6,11\n12,13,4\n16,4,6\n3,4,11\n5,14,12\n16,18,7\n11,17,13\n9,7,4\n17,13,3\n13,15,5\n8,17,13\n14,8,20\n2,8,14\n15,3,16\n12,19,6\n7,7,19\n6,7,19\n11,10,19\n5,19,9\n7,5,5\n7,9,17\n7,8,17\n16,6,8\n14,16,18\n16,10,7\n4,15,12\n13,20,11\n10,15,4\n14,17,13\n2,15,14\n10,15,17\n7,9,1\n10,17,11\n16,6,13\n17,16,15\n13,17,11\n17,14,5\n7,11,4\n13,5,7\n7,6,16\n14,9,1\n16,15,13\n15,5,14\n3,11,6"
  in  "Example":string="2,2,2\n1,2,2\n3,2,2\n2,1,2\n2,3,2\n2,2,1\n2,2,3\n2,2,4\n2,2,6\n1,2,5\n3,2,5\n2,1,5\n2,3,5"
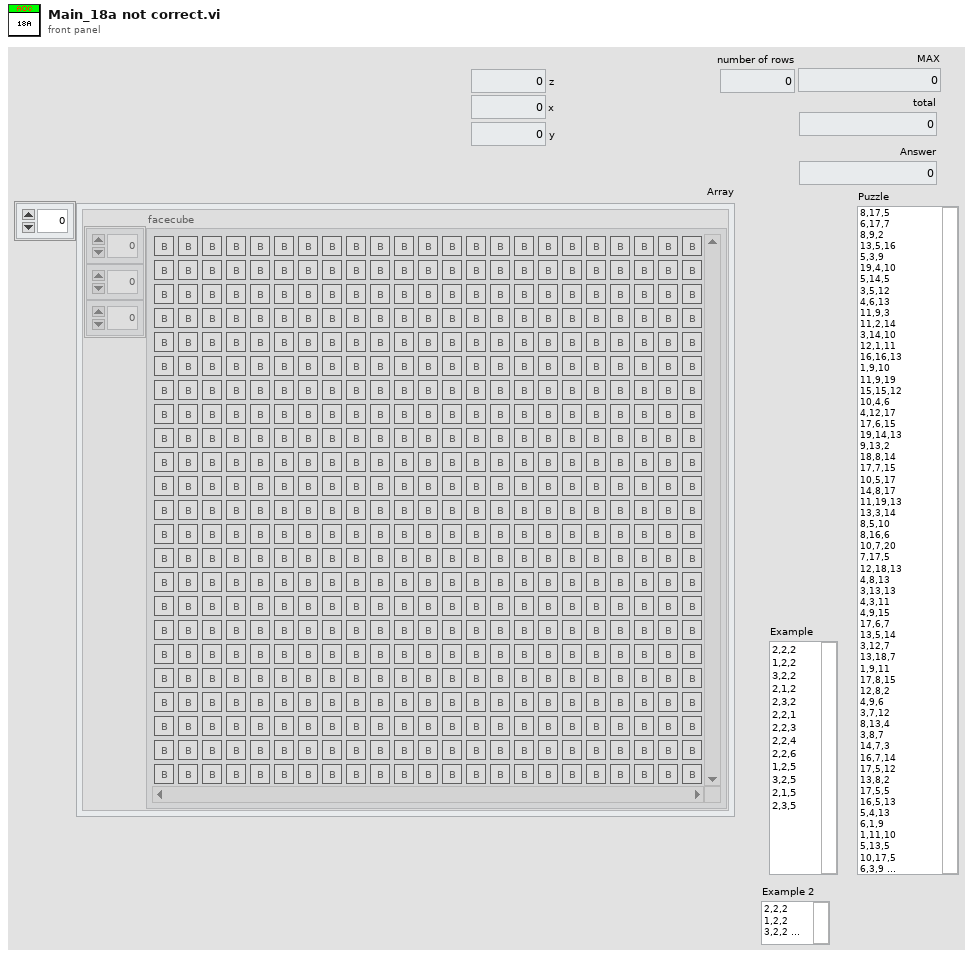
[diagram p1: front panel]
types:
  T1 = typedef "RB ENUM_face state.ctl" = enum32{"Blank", "Exposed", "Faced"}
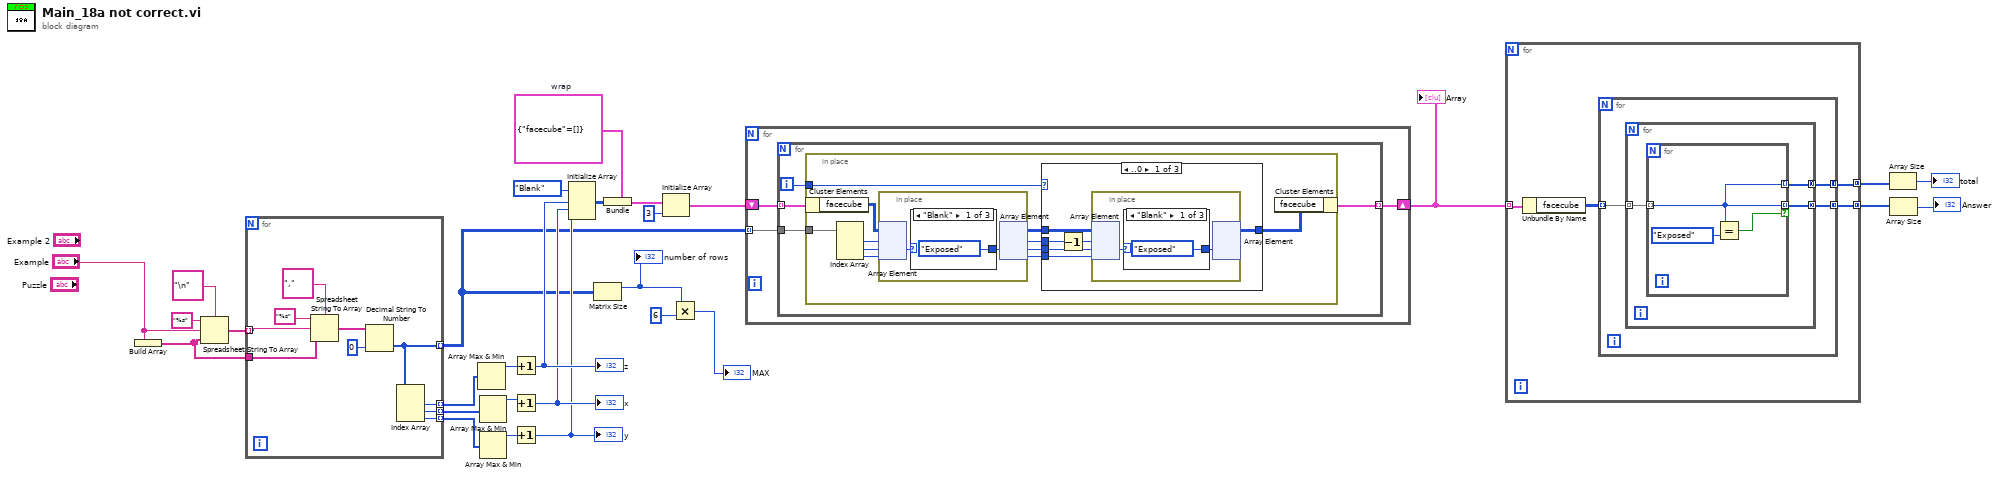
[diagram p0: block diagram]
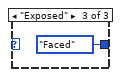
[diagram p3: hidden frame]
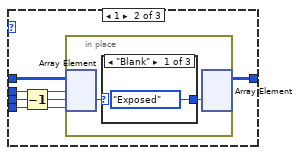
[diagram p4: hidden frame]
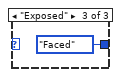
[diagram p6: hidden frame]
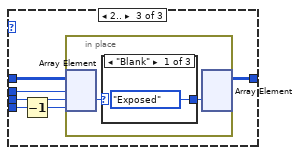
[diagram p7: hidden frame]
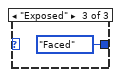
[diagram p9: hidden frame]
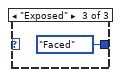
[diagram p11: hidden frame]
diagram:
  w11 = cluster{"facecube":T1[][][]} {"facecube"=[]}  # wrap
  n1 = Build Array("Example") -> (w26:string[])
  n2 = Spreadsheet String To Array(delimiter (Tab)="\n", format string="%s", spreadsheet string="Example", array type (2D Dbl)=w26) -> (array=w27:string[])
  n3 = for {
    tunnel: w27 -> [w36] mode=indexing
    tunnel: w26 -> [w37]
    tunnel: [w33] -> w7 mode=indexing
    tunnel: [w32] -> w25 mode=indexing
    tunnel: [w31] -> w24 mode=indexing
    tunnel: [w30] -> w23 mode=indexing
    n4 = Spreadsheet String To Array(delimiter (Tab)=",", format string="%s", spreadsheet string=w36, array type (2D Dbl)=w37) -> (array=w34:string[])
    n5 = Decimal String To Number(string=w34, default (0L)=0 ("default (0 I32)")) -> (number=w33:i32[])  [unwired: 1 in, 1 out]
    n6 = Index Array(array=w33) -> (element #1=w32:i32, element #2=w31:i32, element #3=w30:i32)  [unwired: 3 in]
  }
  n7 = Array Max & Min(array=w25) -> (max value=w22:i32)  [unwired: 3 out]
  n8 = Array Max & Min(array=w24) -> (max value=w21:i32)  [unwired: 3 out]
  n9 = Array Max & Min(array=w23) -> (max value=w20:i32)  [unwired: 3 out]
  n10 = Increment(x=w22) -> (x+1=w18:i32)
  "z" <- w18
  n11 = Increment(x=w21) -> (x+1=w17:i32)
  "x" <- w17
  n12 = Increment(x=w20) -> (x+1=w16:i32)
  "y" <- w16
  n13 = Initialize Array(RB_ENUM_face_state."Blank" ("Radio Buttons"), w18, w17, w16) -> (w15:T1[][][])
  n14 = Matrix Size(0:w7) -> (1:w4:i32)  [unwired: 1 out]
  "number of rows" <- w4
  n15 = Bundle(cluster=w11, "facecube"=w15) -> (w14:cluster{"facecube":T1[][][]})
  n16 = Initialize Array(w14, 3 ("dimension size")) -> (w12:cluster{"facecube":T1[][][]}[])
  n17 = Multiply(x=w4, y=6) -> (x*y=→"MAX":i32)
  n18 = for {
    shift-right: [w40] -> w10
    shift-left: w12 -> [w41]
    tunnel: w7 -> [w42] mode=indexing
    n19 = for {
      tunnel: w42 -> [w45]
      tunnel: w41 -> [w46] mode=indexing
      tunnel: [w44] -> w40 mode=indexing
      i -> [w43]
      n20 = in-place {
        in-place-border: w45 -> [w57]
        in-place-border: w43 -> [w47]
        n21 = in-place-cluster #1(w46) -> ("facecube"=w56:T1[][][])
        n22 = Index Array(array=w57) -> (element #1=w55:i32, element #2=w54:i32, element #3=w53:i32)  [unwired: 3 in]
        n23 = in-place {
          n24 = in-place-array #2(w56, w55, w54, w53) -> (w92:T1)
          n25 = case shown="\"Blank\"" w92 {
            selector: w92 -> [_ w94 _]
            tunnel: [RB_ENUM_face_state."Exposed" ("element") w94 RB_ENUM_face_state."Faced" ("element")] -> w91
            frame "Blank" {
            }
            frame "Faced" {
            }
            frame "Exposed" {
            }
          }
          n26 = in-place-array #2(w91) -> (w52:T1[][][], w51:i32, w49:i32, w48:i32)
        }
        n27 = case shown="..0" w47 {
          tunnel: w52 -> [w63 w74 w85]
          tunnel: w51 -> [w62 w70 w82]
          tunnel: [w60 w73 w84] -> w50
          tunnel: w49 -> [w59 w72 w81]
          tunnel: w48 -> [w58 w71 w83]
          frame ..0 {
            n28 = Decrement(x=w62) -> (x-1=w61:i32)
            n29 = in-place {
              n30 = in-place-array #3(w63, w61, w59, w58) -> (w65:T1)
              n31 = case shown="\"Blank\"" w65 {
                selector: w65 -> [_ w67 _]
                tunnel: [RB_ENUM_face_state."Exposed" ("element") w67 RB_ENUM_face_state."Faced" ("element")] -> w64
                frame "Blank" {
                }
                frame "Faced" {
                }
                frame "Exposed" {
                }
              }
              n32 = in-place-array #3(w64) -> (w60:T1[][][])  [unwired: 3 out]
            }
          }
          frame 1 {
            n33 = Decrement(x=w72) -> (x-1=w69:i32)
            n34 = in-place {
              n35 = in-place-array #4(w74, w70, w69, w71) -> (w76:T1)
              n36 = case shown="\"Blank\"" w76 {
                selector: w76 -> [_ w78 _]
                tunnel: [RB_ENUM_face_state."Exposed" ("element") w78 RB_ENUM_face_state."Faced" ("element")] -> w75
                frame "Blank" {
                }
                frame "Faced" {
                }
                frame "Exposed" {
                }
              }
              n37 = in-place-array #4(w75) -> (w73:T1[][][])  [unwired: 3 out]
            }
          }
          frame 2.. {
            n38 = Decrement(x=w83) -> (x-1=w80:i32)
            n39 = in-place {
              n40 = in-place-array #5(w85, w82, w81, w80) -> (w87:T1)
              n41 = case shown="\"Blank\"" w87 {
                selector: w87 -> [_ w89 _]
                tunnel: [RB_ENUM_face_state."Exposed" ("element") w89 RB_ENUM_face_state."Faced" ("element")] -> w86
                frame "Blank" {
                }
                frame "Faced" {
                }
                frame "Exposed" {
                }
              }
              n42 = in-place-array #5(w86) -> (w84:T1[][][])  [unwired: 3 out]
            }
          }
        }
        n43 = in-place-cluster #1("facecube"=w50) -> (w44:cluster{"facecube":T1[][][]})
      }
    }
  }
  "Array" <- w10
  n44 = for {
    tunnel: w10 -> [w99] mode=indexing
    tunnel: [w97] -> w9 mode=concatenating
    tunnel: [w96] -> w6 mode=concatenating
    n45 = Unbundle By Name(w99) -> ("facecube"=w98:T1[][][])
    n46 = for {
      tunnel: w98 -> [w102] mode=indexing
      tunnel: [w101] -> w97 mode=concatenating
      tunnel: [w100] -> w96 mode=concatenating
      n47 = for {
        tunnel: w102 -> [w105] mode=indexing
        tunnel: [w104] -> w101 mode=concatenating
        tunnel: [w103] -> w100 mode=concatenating
        n48 = for {
          tunnel: w105 -> [w106] mode=indexing
          tunnel: [w106] -> w104 mode=indexing if=w107
          tunnel: [w106] -> w103 mode=indexing
          n49 = Equal?(x=w106, y=RB_ENUM_face_state."Exposed") -> (x = y?=w107:bool)
        }
      }
    }
  }
  n50 = Array Size(array=w6) -> (size(s)=→"total":i32)
  n51 = Array Size(array=w9) -> (size(s)=→"Answer":i32)
